vi "Flatten.vi"(6 "Indent":i32, 7 "ILinked List in":refnum<class "ILinked List.lvclass">, 8 "error in (no error)":errorcluster, 9 "Child IDs":string[](array[string]), 11 "IPersist in":refnum<class "IPersist.lvclass">) -> (0 "error out":errorcluster, 1 "Flattened Linked List":string[](array[string]), 3 "IPersist out":refnum<class "IPersist.lvclass">, 5 "ILinked List out":refnum<class "ILinked List.lvclass">)   [LabVIEW 2020, in "Linked Lists.lvlib" / "ILinked List.lvclass"]
uses:
  <vilib>/gpm_packages/@cs/linked-list/Source/Linked List/ILinkedList/ILinked List.lvclass
  <vilib>/gpm_packages/@cs/persistence/source/IPersist/IPersist.lvclass
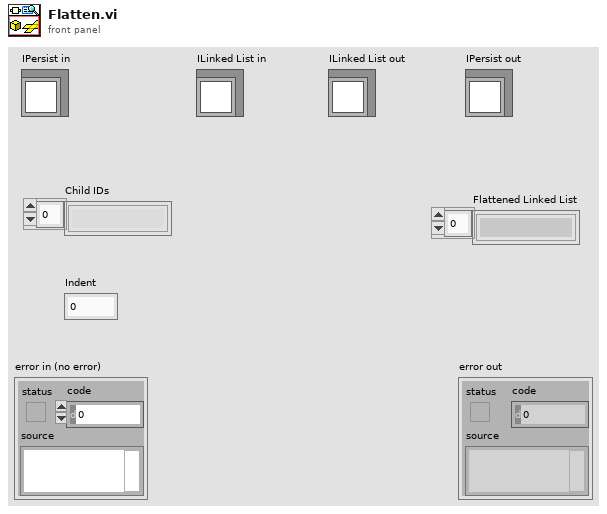
[diagram p1: front panel]
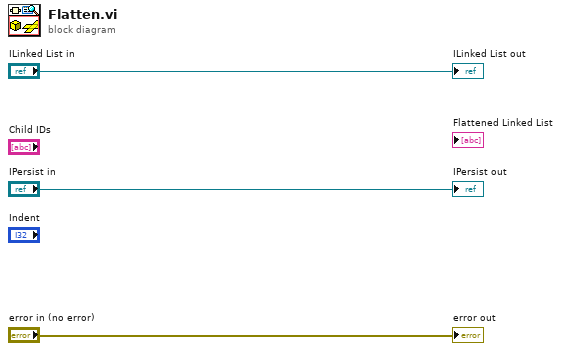
[diagram p0: block diagram]
diagram:
  "error out" <- "error in (no error)"
  "ILinked List out" <- "ILinked List in"
  "IPersist out" <- "IPersist in"
